vi "set imu config to defaults.vi"(8 "error in (no error)":errorcluster, 11 "conf":T1={"accel_fsr"=0, "gyro_fsr"=0, "gyro_dlpf"=0, "accel_dlpf"=0, "enable_magnetometer"=0, "dmp_sample_rate"=0, "orientation"=136, "compass_mix_factor"=0, "dmp_interrupt_priority"=0, "show_warnings"=0} {"accel_fsr" items=["A_FSR_2G", "A_FSR_4G", "A_FSR_8G", "A_FSR_16G"]; "gyro_fsr" items=["G_FSR_250DPS", "G_FSR_500DPS", "G_FSR_1000DPS", "G_FSR_2000DPS"]; "gyro_dlpf" items=["GYRO_DLPF_OFF", "GYRO_DLPF_184", "GYRO_DLPF_92", "GYRO_DLPF_41", "GYRO_DLPF_20", "GYRO_DLPF_10", "GYRO_DLPF_5"]; "accel_dlpf" items=["ACCEL_DLPF_OFF", "ACCEL_DLPF_184", "ACCEL_DLPF_92", "ACCEL_DLPF_41", "ACCEL_DLPF_20", "ACCEL_DLPF_10", "ACCEL_DLPF_5"]; "orientation" items=["ORIENTATION_Z_UP"=136, "ORIENTATION_Z_DOWN"=396, "ORIENTATION_X_UP"=14, "ORIENTATION_X_DOWN"=266, "ORIENTATION_Y_UP"=112, "ORIENTATION_Y_DOWN"=336]}) -> (0 "error out":errorcluster, 2 "function return":i32, 3 "conf out":T1={"accel_fsr"=0, "gyro_fsr"=0, "gyro_dlpf"=0, "accel_dlpf"=0, "enable_magnetometer"=0, "dmp_sample_rate"=0, "orientation"=136, "compass_mix_factor"=0, "dmp_interrupt_priority"=0, "show_warnings"=0} {"accel_fsr" items=["A_FSR_2G", "A_FSR_4G", "A_FSR_8G", "A_FSR_16G"]; "gyro_fsr" items=["G_FSR_250DPS", "G_FSR_500DPS", "G_FSR_1000DPS", "G_FSR_2000DPS"]; "gyro_dlpf" items=["GYRO_DLPF_OFF", "GYRO_DLPF_184", "GYRO_DLPF_92", "GYRO_DLPF_41", "GYRO_DLPF_20", "GYRO_DLPF_10", "GYRO_DLPF_5"]; "accel_dlpf" items=["ACCEL_DLPF_OFF", "ACCEL_DLPF_184", "ACCEL_DLPF_92", "ACCEL_DLPF_41", "ACCEL_DLPF_20", "ACCEL_DLPF_10", "ACCEL_DLPF_5"]; "orientation" items=["ORIENTATION_Z_UP"=136, "ORIENTATION_Z_DOWN"=396, "ORIENTATION_X_UP"=14, "ORIENTATION_X_DOWN"=266, "ORIENTATION_Y_UP"=112, "ORIENTATION_Y_DOWN"=336]})   [LabVIEW 2014, in "test_IMU.lvlib"]
doc: "int set_imu_config_to_defaults(imu_config_t *conf);"
uses:
  <userlib>/test_IMU/test_IMU.lvlib
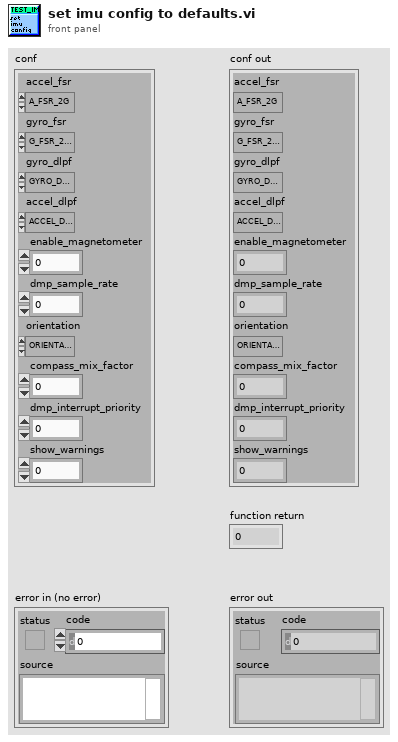
[diagram p1: front panel]
types:
  T1 = cluster{"accel_fsr":u32, "gyro_fsr":u32, "gyro_dlpf":u32, "accel_dlpf":u32, "enable_magnetometer":i32, "dmp_sample_rate":i32, "orientation":u32, "compass_mix_factor":i32, "dmp_interrupt_priority":i32, "show_warnings":i32}
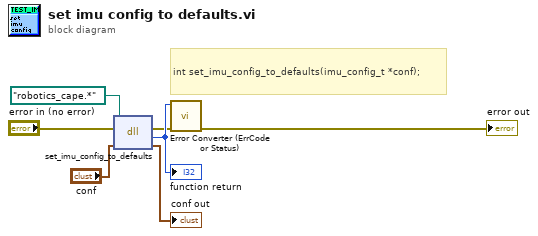
[diagram p0: block diagram]
diagram:
  # "int set_imu_config_to_defaults(imu_config_t *conf);"
  n1 = dll-call lib="C:/Users/ktalke/Documents/Updated Header File/6.18.16/Compiled SO -schroot/robotics_cape.so" fn="set_imu_config_to_defaults"(path in=path "robotics_cape.*", error in="error in (no error)", "conf"="conf") -> (error out=w3:errorcluster, "return type"=w7:i32, "conf"=→"conf out":T1)  [unwired: 1 in, 1 out]
  "function return" <- w7
  n2 = call <userlib>:"Error Converter (ErrCode or Status).vi"("error in (no error)"=w3, "error code"=w7) -> ("error out"=→"error out":errorcluster)  [unwired: 9 in]
